vi "Comm - Send SMS.vi"(8 "error in (no error)":errorcluster, 11 "url":string="https://www.etracker.cc/mes/mesbulk.aspx?user=mktest76&pass=cameron76spt&type=5&to=6584186990&from=SRTRS&text=65B052A05761&servid=MES01") -> (0 "error out":errorcluster, 3 "MobileNo, MessageRefNo, StatusId":string[](array[string]))   [LabVIEW 2013]
uses:
  <vilib>/httpClient/POSTBuffer.vi
  <vilib>/httpClient/LabVIEWHTTPClient.lvlib
panel:
  in  "String":string="°e RaW"
  out "body":string
  out "headers":string
  # "UCS2 - Swapped Byte"
  # "https://www.etracker.cc/mes/mesbulk.aspx?user=mktest76&pass=cameron76spt&type=5&to=6584186990&from=SRTRS&text=65B052A05761&servid=MES01"
  # "https://www.etracker.cc/mes/mesbulk.aspx?user=mktest76&pass=cameron76spt&type=5&to=6584186990&from=SRTRS&text=005300520054005200530053004D00530053007400720069006E006700310053004D00530053007400720069006E00670032005B003300340035003600370038003900310030002C00310031005D0053004D00530053007400720069006E006700310032002E&servid=MES01"
  # "https://www.etracker.cc/mes/mesbulk.aspx?user=mktest76&pass=cameron76spt&type=5&to=6584186990&from=SRTRS&text=65B052A05761&servid=MES01"
  # "https://www.etracker.cc/mes/mesbulk.aspx?user=mktest76&pass=cameron76spt&type=5&to=6584186990&from=SRTRS&text=B065A0526157&servid=MES01"
  # "https://www.etracker.cc/mes/mesbulk.aspx?user=mktest76&pass=cameron76spt&type=5&to=6584186990&from=SRTRS&text=65B052A05761&servid=MES01"
  # "https://www.etracker.cc/mes/mesbulk.aspx?user=mktest76&pass=cameron76spt&type=0&to=6584186990&from=SRTRS&text=SMS+forward+test+from+SRTRS&servid=MES01"
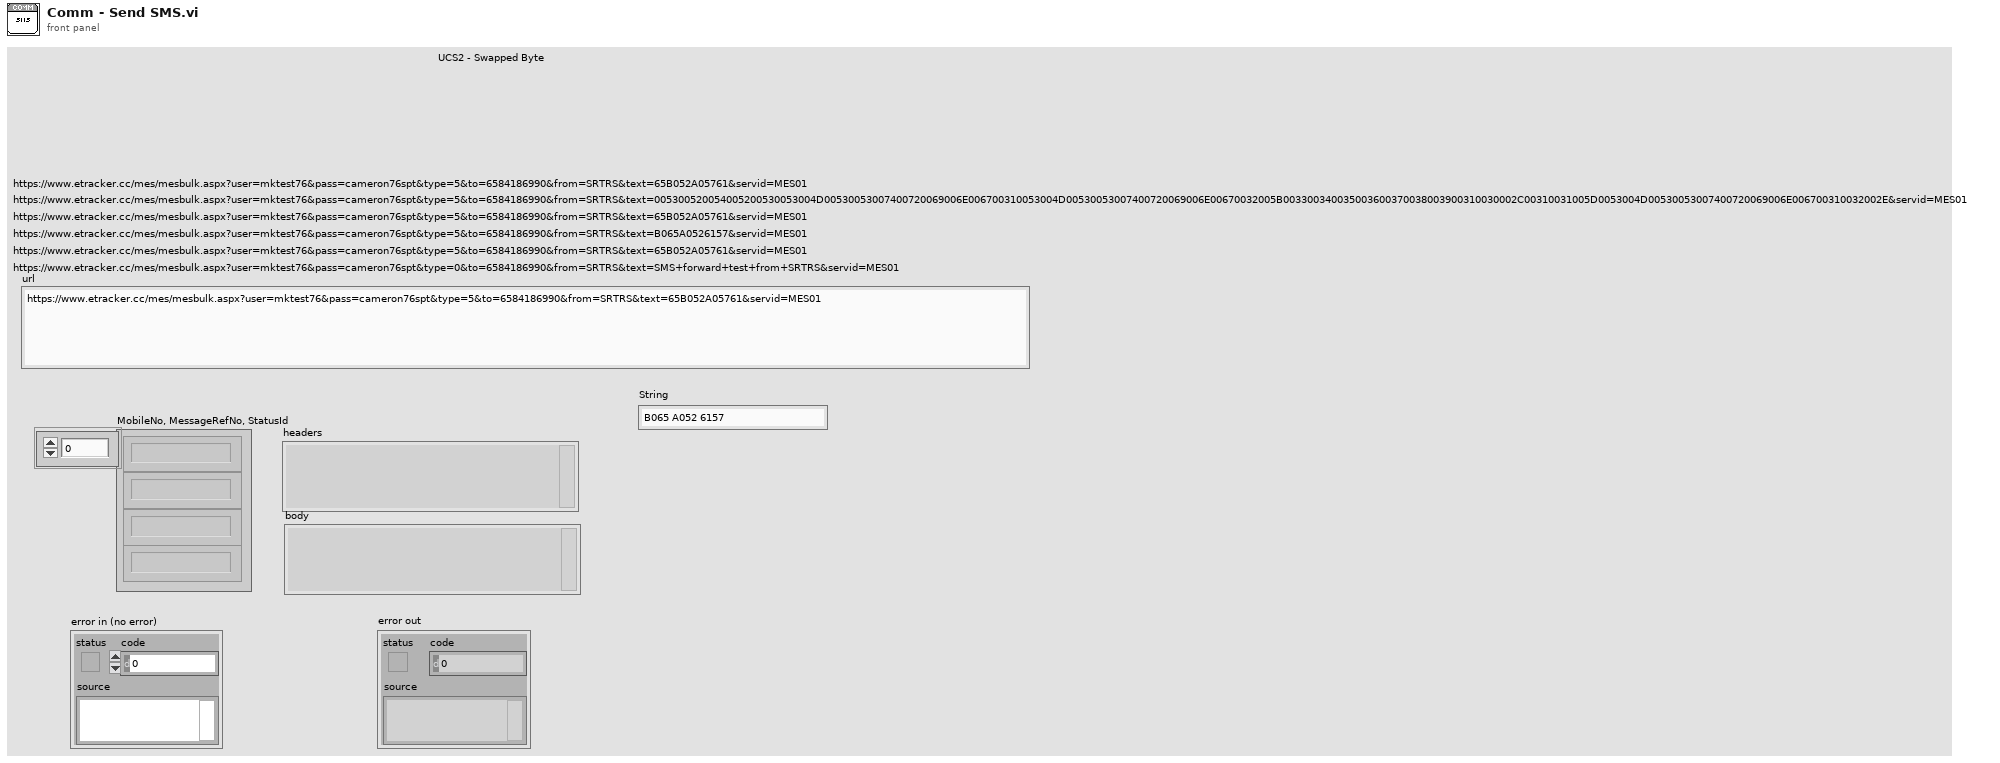
[diagram p1: front panel]
types:
  T1 = typedef "LabVIEWHTTPClient.lvlib/ClientHandle.ctl" = refnum<k1>
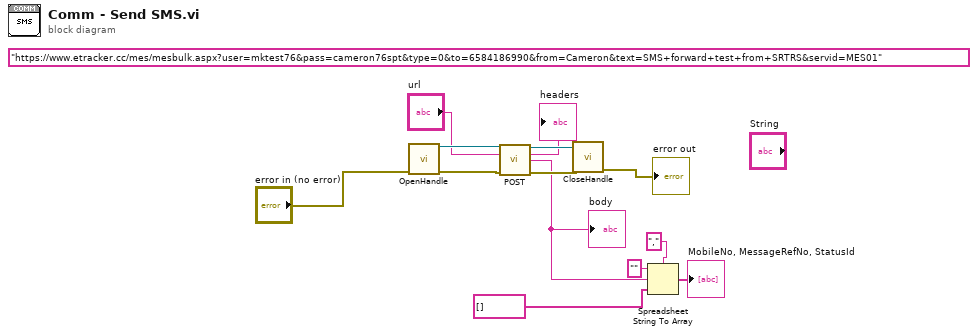
[diagram p0: block diagram]
diagram:
  (unwired) "https://www.etracker.cc/mes/mesbulk.aspx?user=mktest76&pass=cameron76spt&type=0&to=6584186990&from=Cameron&text=SMS+forward+test+from+SRTRS&servid=MES01" ("url")
  n1 = call <vilib>:"OpenHandle.vi"("error in (no error)"="error in (no error)") -> ("client handle out"=w13:T1, "error out"=w12:errorcluster)  [unwired: 13 in]
  n2 = call-poly <vilib>:"POST.vi"("client handle"=w13, "url"="url", "error in (no error)"=w12) -> ("client handle out"=w11:T1, "headers"=→"headers":string, "body"=w6:string, "error out"=w10:errorcluster)  [unwired: 9 in]
  "body" <- w6
  n3 = call <vilib>:"CloseHandle.vi"("client handle"=w11, "error in (no error)"=w10) -> ("error out"=→"error out":errorcluster)  [unwired: 13 in]
  n4 = Spreadsheet String To Array(delimiter (Tab)=",", format string="", spreadsheet string=w6, array type (2D Dbl)=string[] []) -> (array=→"MobileNo, MessageRefNo, StatusId":string[])
